vi "Display Custom Shortcut Menu.vi"(8 "error in (no error)":errorcluster, 10 "MenuRef":refnum<k9>, 11 "IControlShortcutMenu In":refnum<class "IControlShortcutMenu.lvclass">) -> (0 "error out":errorcluster, 2 "Discarded?":bool, 3 "IControlShortcutMenu Out":refnum<class "IControlShortcutMenu.lvclass">)   [LabVIEW 2015, in "ActorEvents.lvlib" / "IControlShortcutMenu.lvclass"]
uses:
  IControlShortcutMenu.lvclass
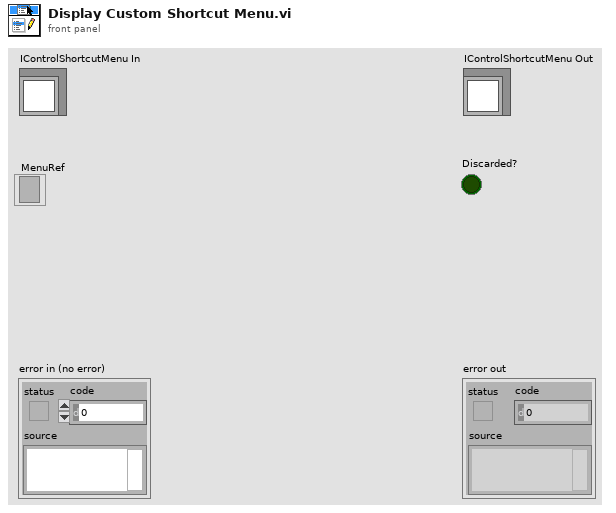
[diagram p1: front panel]
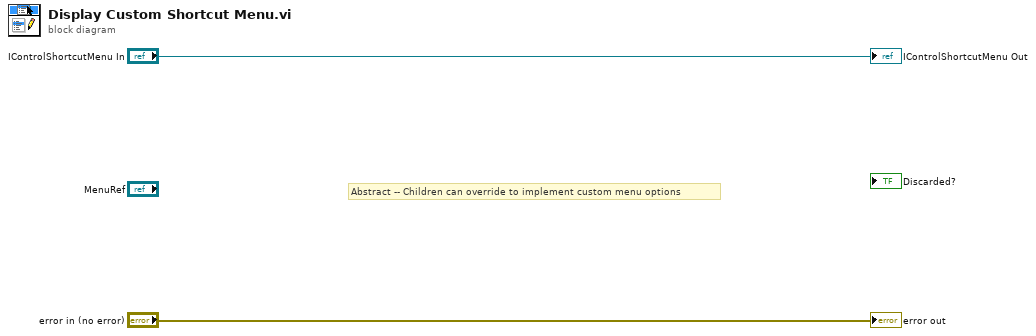
[diagram p0: block diagram]
diagram:
  # "Abstract -- Children can override to implement custom menu options"
  "error out" <- "error in (no error)"
  "IControlShortcutMenu Out" <- "IControlShortcutMenu In"
